vi "CMD_01_Set_DAC1.vi"(9 "Input, V":dbl min=-50.0 max=50.0, 11 "VISA resource name":refnum<visa-resource-name>) -> (0 "16bit integer":i16, 3 "VISA resource name out":refnum<visa-resource-name>)   [LabVIEW 2017]
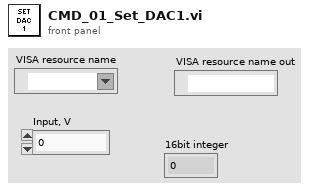
[diagram p1: front panel]
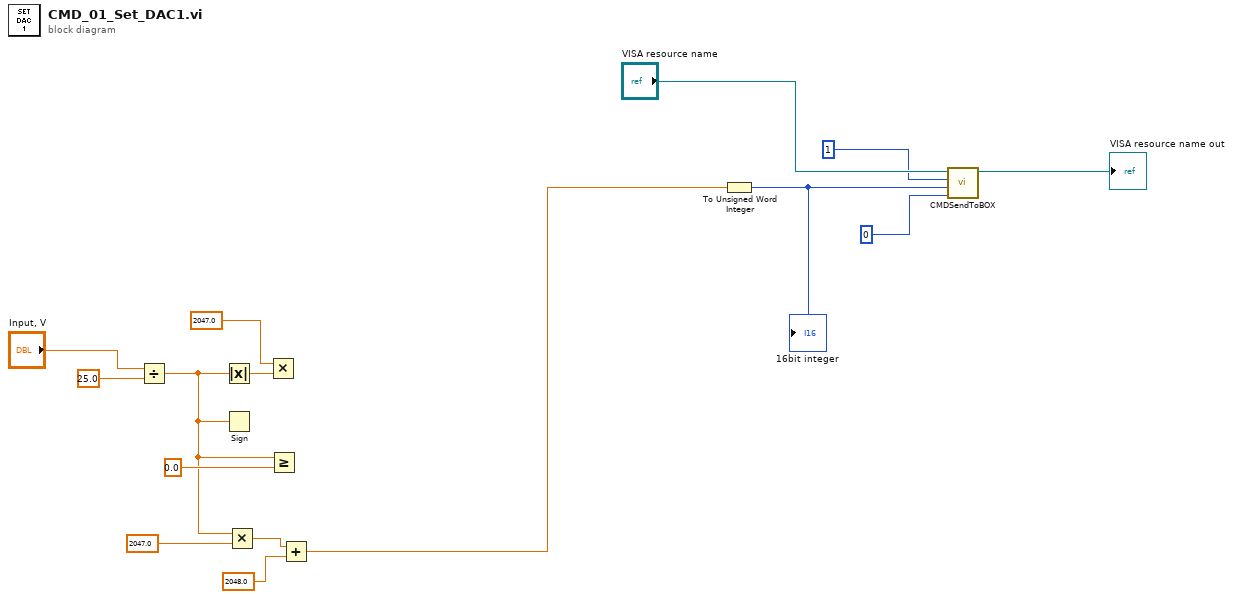
[diagram p0: block diagram]
diagram:
  n1 = Divide(x="Input, V", y=25.0) -> (x/y=w6:dbl)
  n2 = Absolute Value(x=w6) -> (abs(x)=w9:dbl)
  n3 = Sign(1:w6) -> ()  [unwired: 1 out]
  n4 = Multiply(x=w6, y=2047.0) -> (x*y=w4:dbl)
  n5 = Multiply(x=2047.0 ("y"), y=w9) -> ()  [unwired: 1 out]
  n6 = Greater Or Equal?(x=w6, y=0.0) -> ()  [unwired: 1 out]
  n7 = Add(x=w4, y=2048.0) -> (x+y=w1:dbl)
  n8 = To Unsigned Word Integer(number=w1) -> (unsigned 16bit integer=w2:u16)
  "16bit integer" <- w2
  n9 = call "CMDSendToBOX.vi"("arg2"=i16 0, "arg1"=w2, "CMD"=i8 1, "VISA resource name"="VISA resource name") -> ("VISA resource name out"=→"VISA resource name out":refnum<visa-resource-name>)  [unwired: 7 in]
